vi "BuildCall.vi"(7 "PythonConverter_BD in":refnum<class "PyConvBD.lvclass">, 8 "error in":errorcluster, 11 "Control Terminal in":refnum<class "ControlTerminal.lvclass">) -> (0 "error out":errorcluster, 3 "Control Terminal out":refnum<class "ControlTerminal.lvclass">, 5 "PythonConverter_BD out":refnum<class "PyConvBD.lvclass">)   [LabVIEW 2014, in "Raspberry Pi Compatible Compiler for LabVIEW.lvlib" / "ControlTerminal.lvclass"]
uses:
  ControlTerminal.lvclass
  Python/PythonConverter_BD/PyConvBD.lvclass
  Python/PythonConverter_BD/TypeDefs/NodeCall_TD.ctl
  Python/Parsing/ListTypesTD.ctl
  Terminal/Terminal.lvclass
  Python/Parsing/Python Functions.lvlib
  Raspberry Pi Compatible Compiler for LabVIEW.lvlib
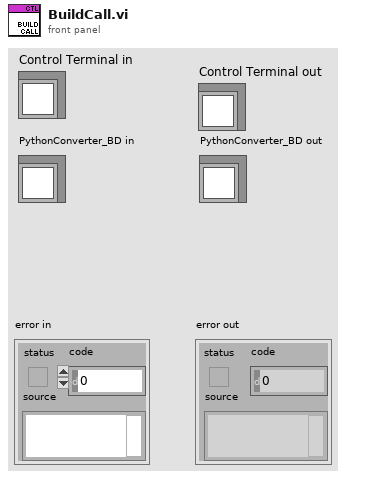
[diagram p1: front panel]
types:
  T1 = typedef "Raspberry Pi Compatible Compiler for LabVIEW.lvlib/NodeCall_TD.ctl" = cluster{"call":string, "collect":string, "Threaded":bool, "branches":string[]}
  T2 = typedef "Raspberry Pi Compatible Compiler for LabVIEW.lvlib/Python Functions.lvlib/ListTypesTD.ctl" = enum16{"list", "tuple", "parameter list", "output list", "return values"}
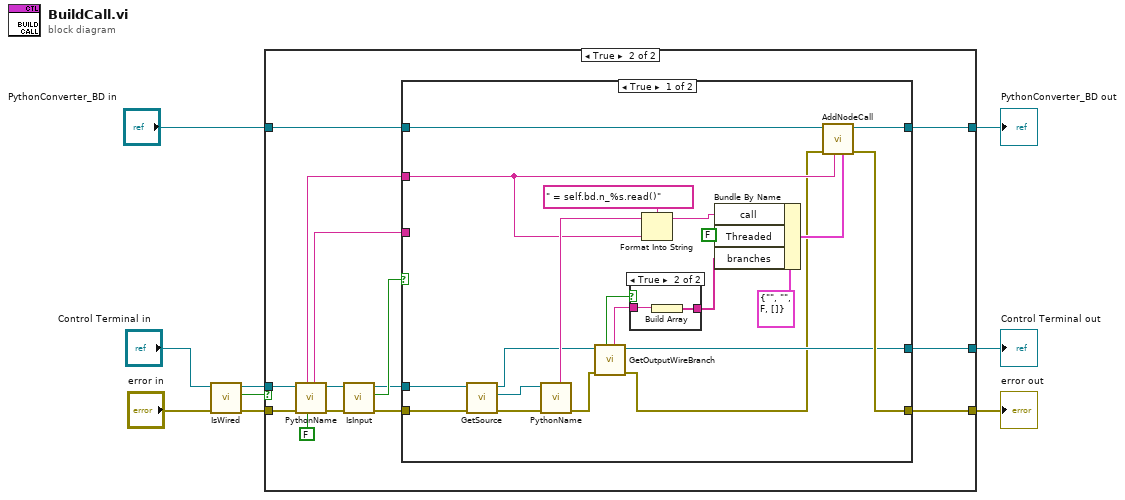
[diagram p0: block diagram]
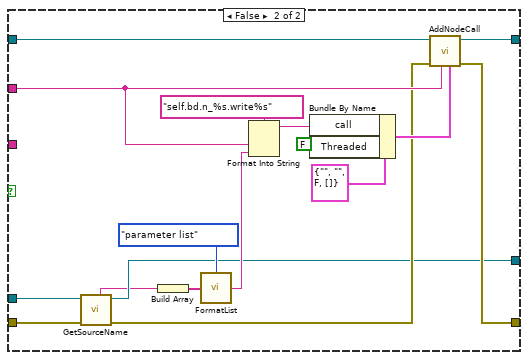
[diagram p4: hidden frame]
diagram:
  n1 = call "IsWired.vi"("error in"="error in", "Terminal in"="Control Terminal in") -> ("error out"=w5:errorcluster, "wired"=w4:bool, "Terminal out"=w3:refnum<class "ControlTerminal.lvclass">)  [unwired: 5 in]
  n2 = case shown="True" w4 {
    tunnel: "PythonConverter_BD in" -> [w12 w26]
    tunnel: [w12 w25] -> w8
    tunnel: [w11 w24] -> w7
    tunnel: [w10 w23] -> w6
    tunnel: w5 -> [w11 w17]
    tunnel: w3 -> [w10 w15]
    frame False {
    }
    frame True {
      n3 = call-dynamic "PythonName.vi"("add self"=FALSE, "error in"=w17, "Terminal in"=w15) -> ("error out"=w19:errorcluster, "Terminal out"=w20:refnum<class "ControlTerminal.lvclass">, "name"=w18:string, "UID"=w13:string)  [unwired: 5 in]
      n4 = call-dynamic "IsInput.vi"("error in"=w19, "ControlTerminal in"=w20) -> ("error out"=w21:errorcluster, "input"=w22:bool, "ControlTerminal out"=w14:refnum<class "ControlTerminal.lvclass">)  [unwired: 5 in]
      n5 = case shown="True" w22 {
        tunnel: w14 -> [w46 w51]
        tunnel: w21 -> [w47 w50]
        tunnel: w18 -> [_ _]
        tunnel: w26 -> [w42 w62]
        tunnel: [w41 w61] -> w24
        tunnel: [w40 w60] -> w25
        tunnel: [w32 w53] -> w23
        tunnel: w13 -> [w38 w59]
        frame True {
          n6 = call "GetSource.vi"("error in"=w47, "Terminal in"=w46) -> ("error out"=w45:errorcluster, "source"=w44:refnum<class "Terminal.lvclass">, "Terminal out"=w33:refnum<class "ControlTerminal.lvclass">)  [unwired: 5 in]
          n7 = call-dynamic "PythonName.vi"("error in"=w45, "Terminal in"=w44) -> ("error out"=w31:errorcluster, "name"=w39:string)  [unwired: 6 in, 2 out]
          n8 = call-dynamic "GetOutputWireBranch.vi"("error in"=w31, "Terminal in"=w33) -> ("error out"=w30:errorcluster, "Terminal out"=w32:refnum<class "ControlTerminal.lvclass">, "branches"=w28:string, "branched"=w29:bool)  [unwired: 4 in]
          n9 = case shown="True" w29 {
            tunnel: w28 -> [_ w49]
            tunnel: [_ w48] -> w27
            frame False {
            }
            frame True {
              n10 = Build Array(w49) -> (w48:string[])
            }
          }
          n11 = Format Into String(format string=" = self.bd.n_%s.read()", initial string=w39, w38) -> (resulting string=w34:string)  [unwired: 1 in, 1 out]
          n12 = Bundle By Name(cluster=T1 {"call"="", "collect"="", "Threaded"=FALSE, "branches"=[]} ("call"), "call"=w34, "Threaded"=FALSE, "branches"=w27) -> (w35:T1)
          n13 = call "AddNodeCall.vi"("call"=w35, "name"=w38, "error in"=w30, "PythonConverter_BD in"=w42) -> ("error out"=w41:errorcluster, "PythonConverter_BD out"=w40:refnum<class "PyConvBD.lvclass">)  [unwired: 4 in]
        }
        frame False {
          n14 = call "GetSourceName.vi"("error in"=w50, "Terminal in"=w51) -> ("error out"=w54:errorcluster, "Terminal out"=w53:refnum<class "ControlTerminal.lvclass">, "source"=w52:string)  [unwired: 5 in]
          n15 = Build Array(w52) -> (w63:string[])
          n16 = call "FormatList.vi"("values"=w63, "type"=ListTypesTD."parameter list") -> ("python object"=w64:string)
          n17 = Format Into String(format string="self.bd.n_%s.write%s", w59, w64) -> (resulting string=w56:string)  [unwired: 2 in, 1 out]
          n18 = Bundle By Name(cluster=T1 {"call"="", "collect"="", "Threaded"=FALSE, "branches"=[]} ("call"), "call"=w56, "Threaded"=FALSE) -> (w55:T1)
          n19 = call "AddNodeCall.vi"("call"=w55, "name"=w59, "error in"=w54, "PythonConverter_BD in"=w62) -> ("error out"=w61:errorcluster, "PythonConverter_BD out"=w60:refnum<class "PyConvBD.lvclass">)  [unwired: 4 in]
        }
      }
    }
  }
  "error out" <- w7
  "Control Terminal out" <- w6
  "PythonConverter_BD out" <- w8
